vi "Process.vi"(8 "error in":errorcluster, 11 "Inst.AH2500":refnum<class "Inst.AH2500.lvclass">) -> (0 "error out":errorcluster, 3 "Inst.AH2500 out":refnum<class "Inst.AH2500.lvclass">)   [LabVIEW 2019, in "Inst.AH2500.lvclass"]
doc: "---------------------------------------------------------------\nJKI State Machine Objects™\nhttp://jki.net/state-machine-objects/\nCopyright (C) 2005-2015, JKI <info@jki.net>\nALL RIGHTS RESERVED"
uses:
  Inst.AH2500.lvclass
  <vilib>/JKI/JKI SMO/SMO/SMO.lvclass
  <userlib>/LevyLab/Instrument Framework/Instrument/Instrument.lvclass
  <userlib>/LevyLab/RemoteControl/RemoteControl/Typedefs/Message--Cluster.ctl
  <userlib>/LevyLab/RemoteControl/RemoteControl/RemoteControl.lvclass
  Typedefs/PrivateEvents--Inst.AH2500.MessageToProcess.ctl
  <userlib>/LevyLab/Instrument Framework/Instrument Types/VSource/Instrument.VSource.lvclass
  <userlib>/LevyLab/Instrument Framework/Instrument/API/Instrument.sendMessageToProcess (string).vi
  C:/Program Files (x86)/National Instruments/LabVIEW 2019/user.lib/LevyLab/Instrument Framework/Instrument Types/VSource/Instrument.VSource.lvclass
  C:/Program Files (x86)/National Instruments/LabVIEW 2019/user.lib/LevyLab/Instrument Framework/Instrument/Instrument.lvclass
  C:/Program Files (x86)/National Instruments/LabVIEW 2019/vi.lib/JKI/JKI SMO/SMO/SMO.lvclass
panel:
  out "Status":string
  out "State History":string
  # "Inst.AH2500"
  # "Inst.AH2500"
  # "For instructions on how to use the JKI State Machine Objects, examples and video tutorials, visit:\nhttp://jki.net/state-machine-objects/\n\nJKI State Machine Objects™\nhttp://jki.net/state-machine-objects/\nCopyright (C) 2005-2015, JKI <info@jki.net>\nALL RIGHTS RESERVED"
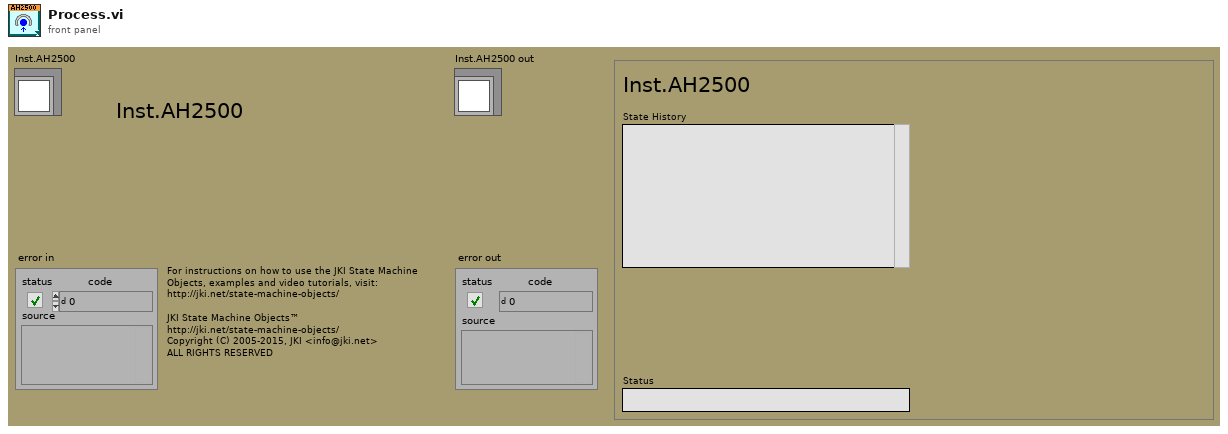
[diagram p1: front panel]
types:
  T1 = enum32{"invalid app kind", "Development System", "Run Time System", "Student Edition", "Embedded LabVIEW", "Evaluation", "Custom"}
  T2 = enum32{"Invalid", "Standard", "Closed", "Hidden", "Minimized", "Maximized"}
  T3 = typedef "RemoteControl.lvclass/Message--Cluster.ctl" = cluster{"Command":string, "Data":variant, "ID":string}
  T4 = typedef "Inst.AH2500.lvclass/PrivateEvents--Inst.AH2500.MessageToProcess.ctl" = cluster{"Message":T5}
  T5 = typedef "RemoteControl.lvlib/RemoteControl.lvclass/Message--Cluster.ctl" = cluster{"Command":string, "Data":variant, "ID":string}
  T6 = cluster{"Core":cluster{"Current VI Reference":refnum<vi>, "Close Panel on Exit?":bool, "Last Error":cluster{"error":errorcluster, "previous state":string, "remaining states":string}, "Shutdown?":bool}, "SelfRef":refnum<class "Inst.AH2500.lvclass">, "Running Step":i32, "sequence":string[], "MessageToProcess":T4}
  T7 = cluster{"Current VI Reference":refnum<vi>, "Close Panel on Exit?":bool, "Last Error":cluster{"error":errorcluster, "previous state":string, "remaining states":string}, "Shutdown?":bool}
  T8 = typedef "smo.lvlib/SMO.lvclass/Protected Events.ctl" = cluster{"StopProcesses":refnum<user-event>, "AbortProcesses":refnum<user-event>, "Config Changed":refnum<user-event>, "Dependency":refnum<user-event>}
  T9 = typedef "Inst.AH2500.lvclass/Inst.AH2500.getAll--Cluster.ctl" = cluster{"capacitance (pF)":dbl, "loss (nS)":dbl, "Vexc (V)":dbl}
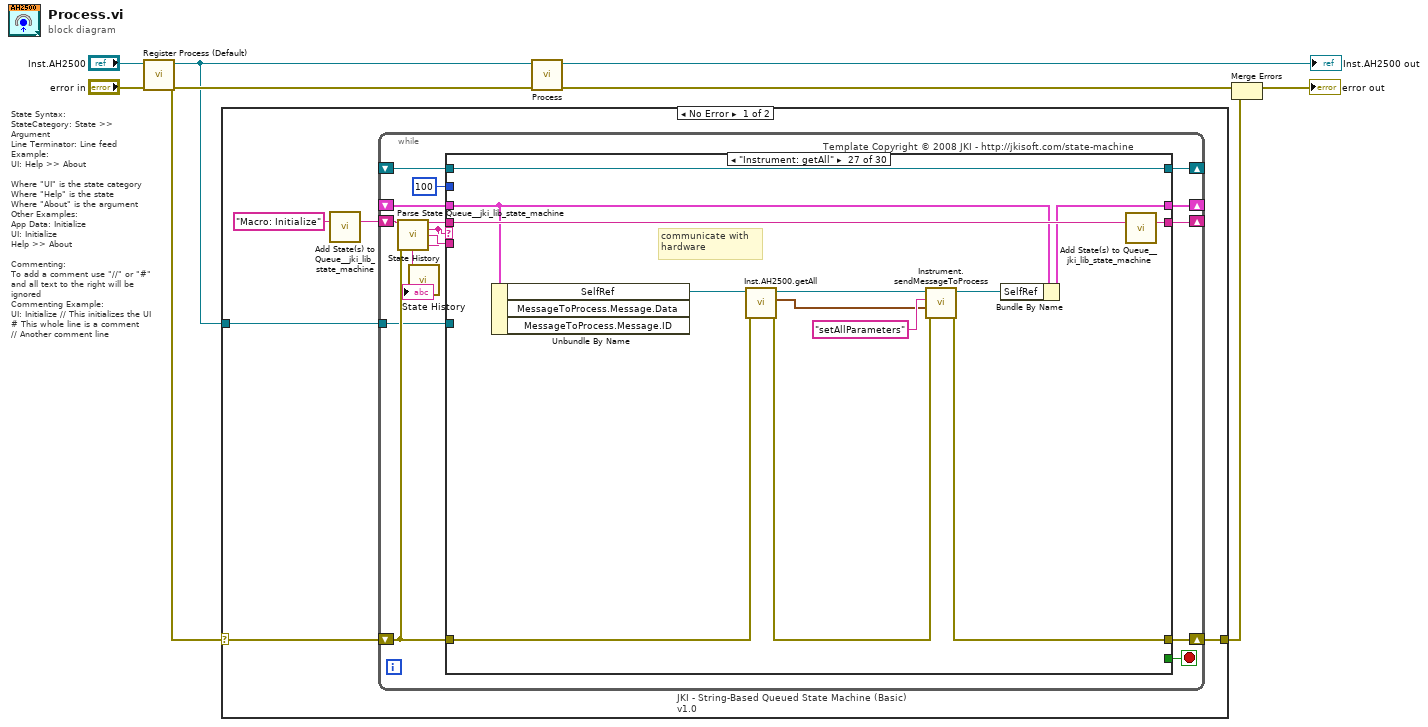
[diagram p0: block diagram]
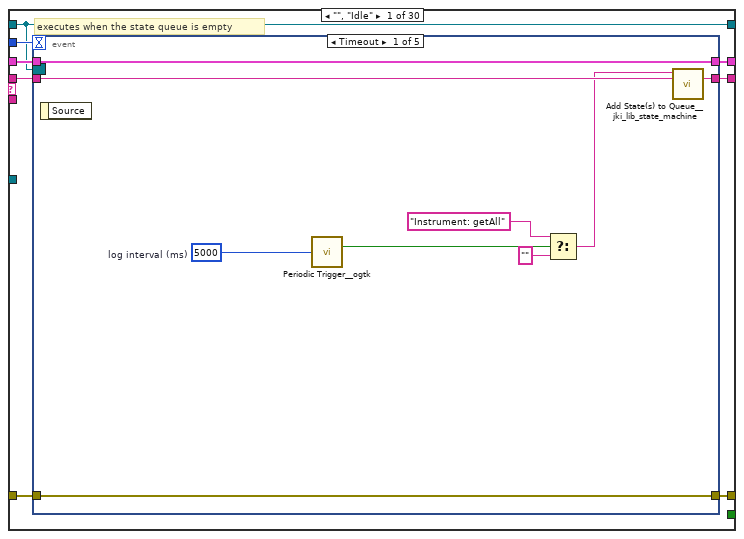
[diagram p2: hidden frame]
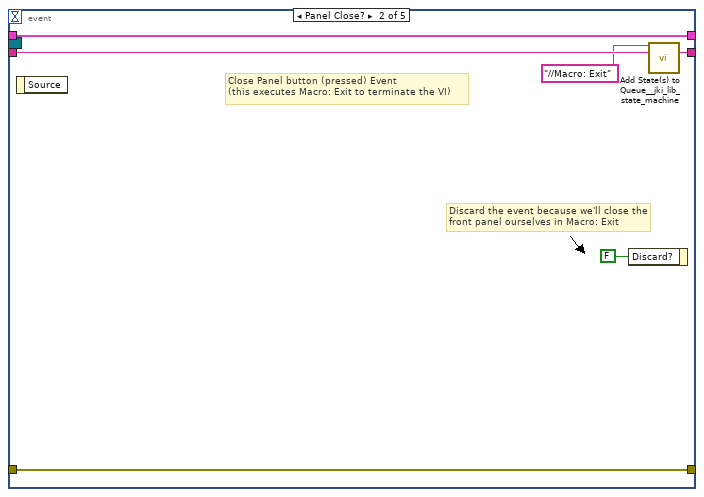
[diagram p3: hidden frame]
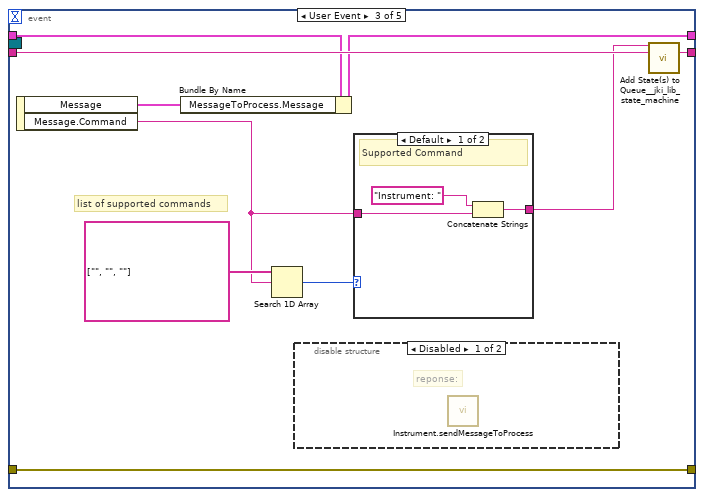
[diagram p4: hidden frame]
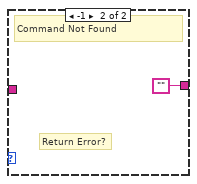
[diagram p6: hidden frame]
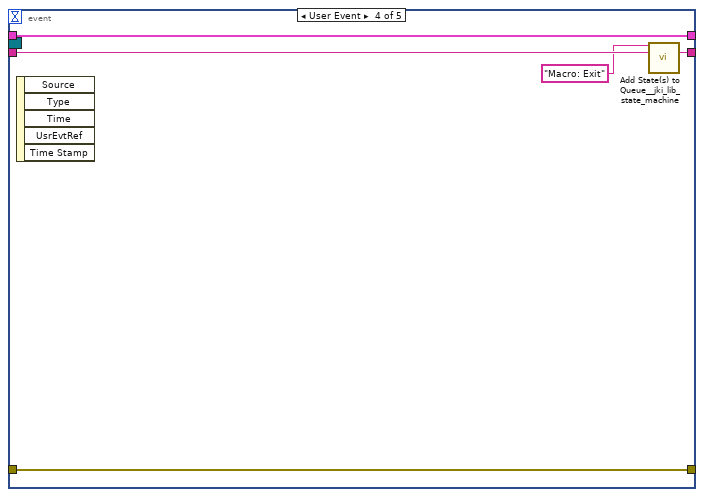
[diagram p7: hidden frame]
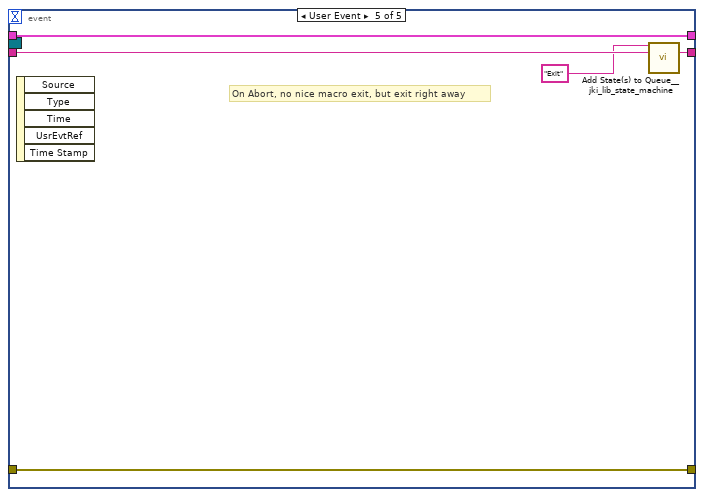
[diagram p8: hidden frame]
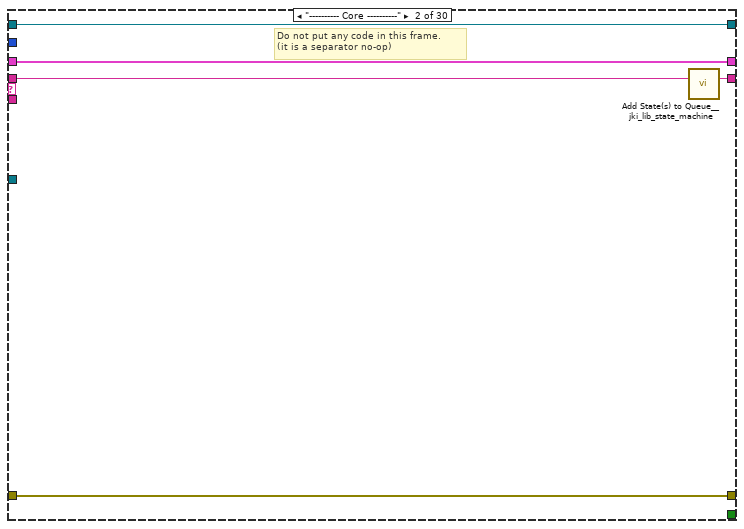
[diagram p9: hidden frame]
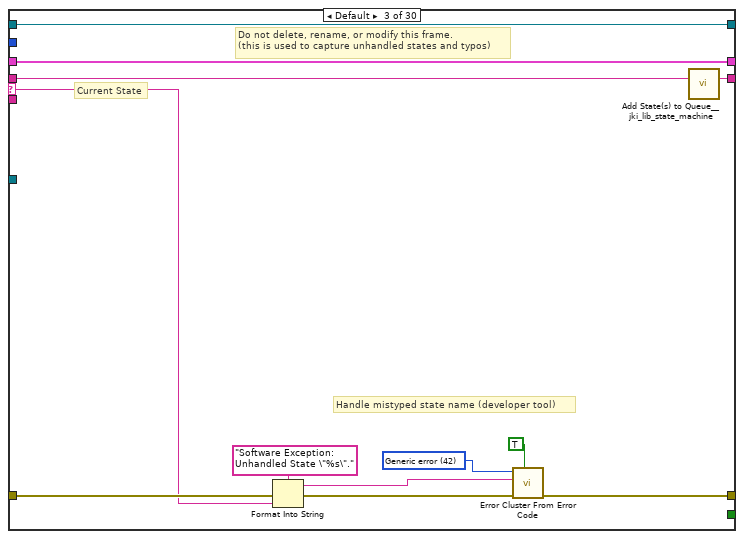
[diagram p10: hidden frame]
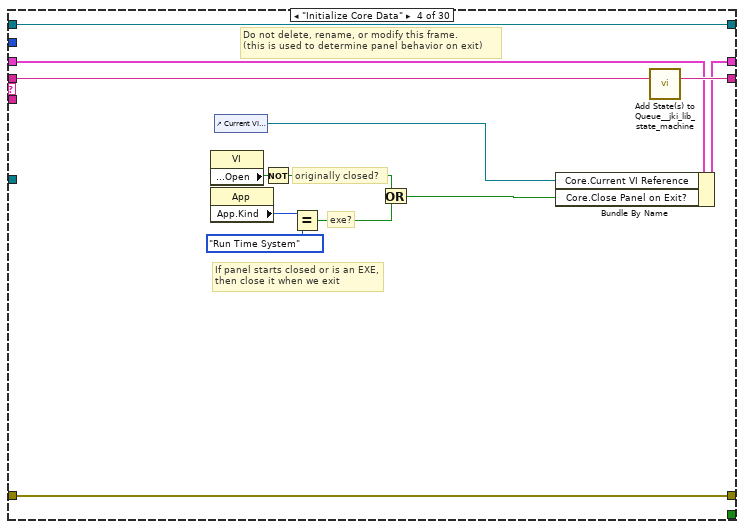
[diagram p11: hidden frame]
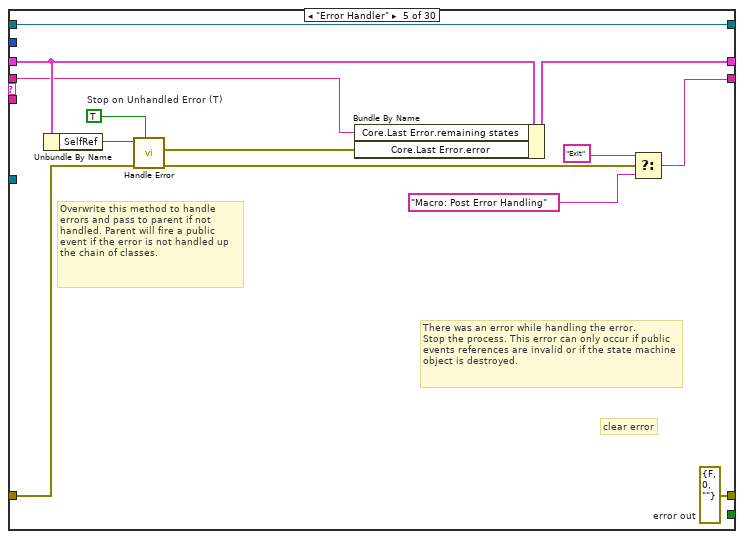
[diagram p12: hidden frame]
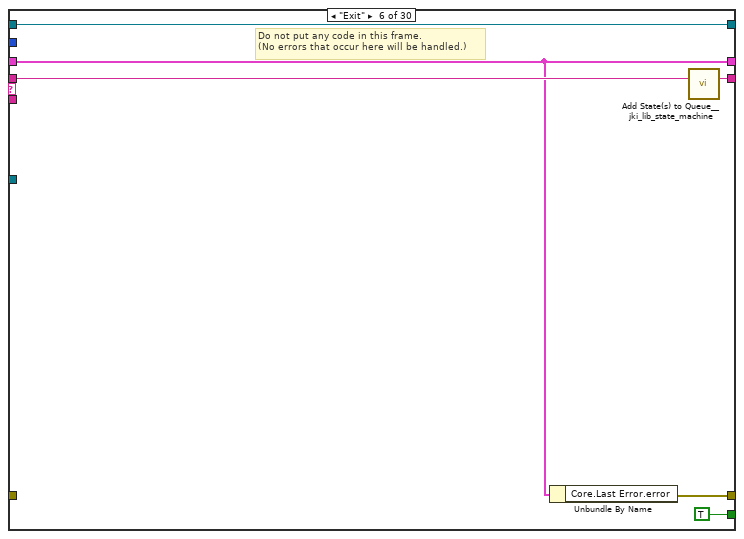
[diagram p13: hidden frame]
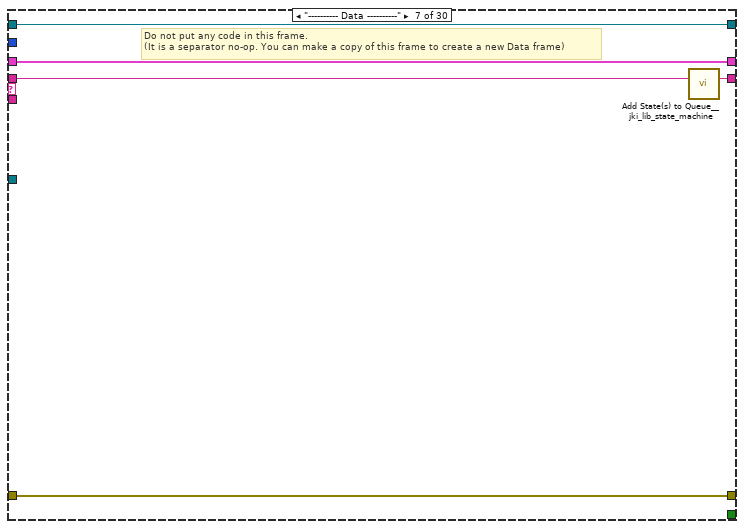
[diagram p14: hidden frame]
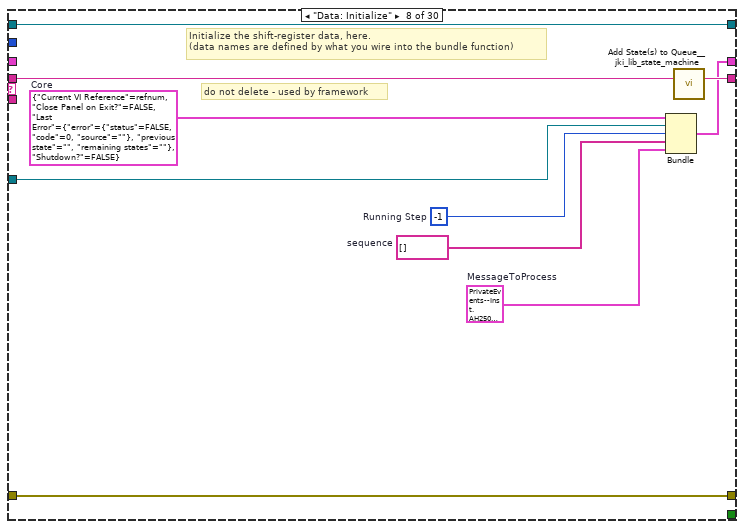
[diagram p15: hidden frame]
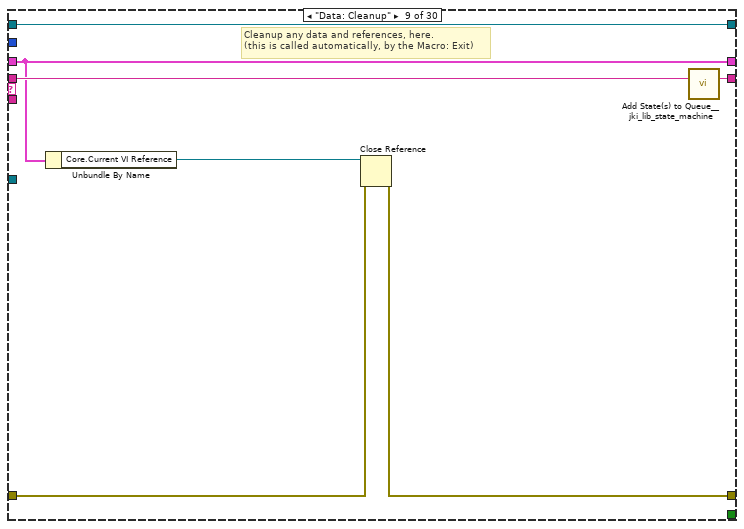
[diagram p16: hidden frame]
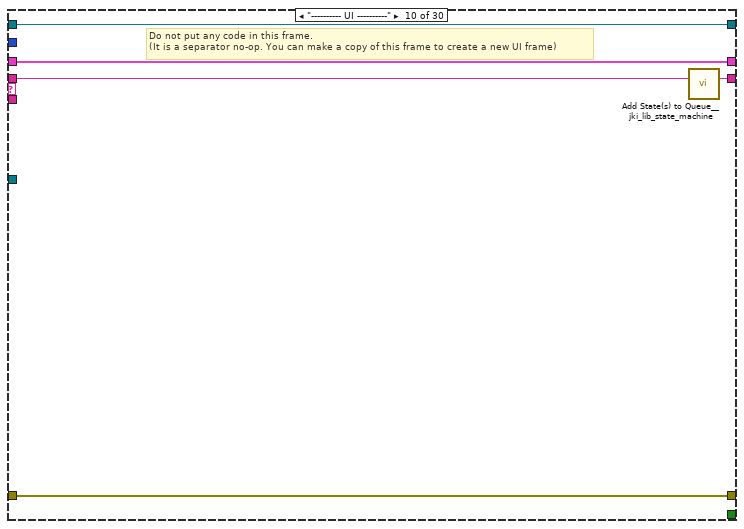
[diagram p17: hidden frame]
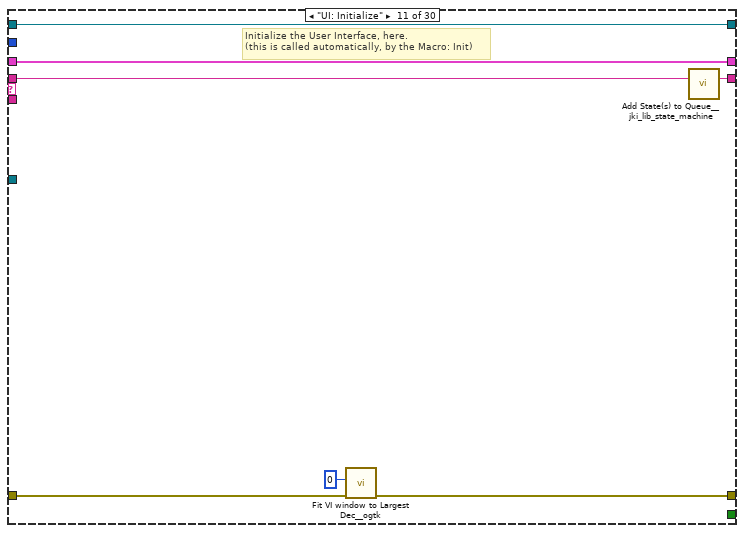
[diagram p18: hidden frame]
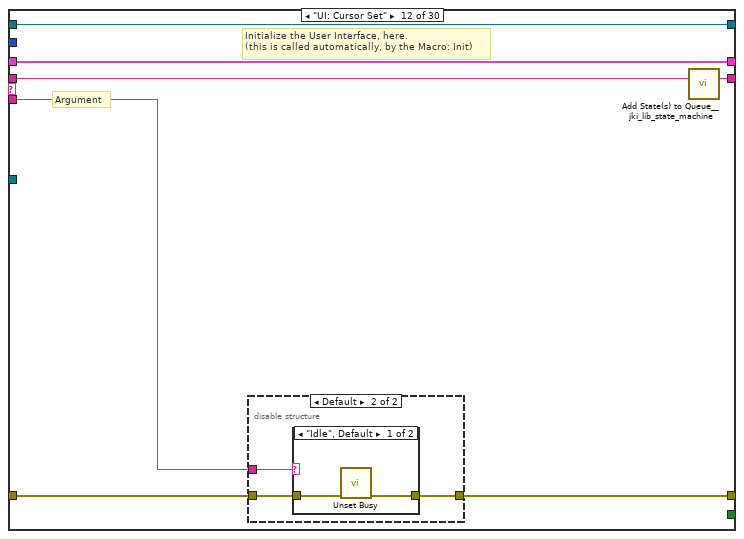
[diagram p19: hidden frame]
diagram:
  # "State Syntax:\nStateCategory: State >> Argument\nLine Terminator: Line feed\nExample:\nUI: Help >> About\n\nWhere \"UI\" is the state category\nWhere \"Help\" is the state\nWhere \"About\" is the argument\nOther Examples:\nApp Data: Initialize\nUI: Initialize\nHelp >> About\n\nCommenting:\nTo add a comment use \"//\" or \"#\" and all text to the right will be ignored\nCommenting Example:\nUI: Initialize // This initializes the UI\n# This whole line is a comment\n// Another comment line"
  n1 = call <vilib>:"Register Process (Default).vi"("error in (no error)"="error in", "SMO"="Inst.AH2500") -> ("error out"=w5:errorcluster, "SelfRef"=w4:refnum<class "Inst.AH2500.lvclass">)  [unwired: 8 in]
  n2 = case shown="No Error" w5 {
    selector: w5 -> [w10 w396]
    tunnel: w4 -> [w11 _]
    tunnel: [w9 w396] -> w1
    frame No Error {
      n3 = call <vilib>:"Add State(s) to Queue__jki_lib_state_machine.vi"("State(s) in (\"\")"="Macro: Initialize") -> ("States Out"=w13:string)  [unwired: 14 in]
      n4 = while "JKI - String-Based Queued State Machine (Basic) v1.0" {
        shift-right: [w22] -> _
        shift-left: _ -> [w21]
        shift-right: [w25] -> w9
        shift-left: w10 -> [w19]
        shift-right: [w24] -> _
        shift-left: w13 -> [w26]
        tunnel: w11 -> [w18]
        shift-right: [w17] -> _
        shift-left: _ -> [w16]
        stop <- w23 stop-if-true
        # "Template Copyright © 2008 JKI - http://jkisoft.com/state-machine"
        n5 = call <vilib>:"Parse State Queue__jki_lib_state_machine.vi"("State Queue"=w26, "Error In (no error)"=w19) -> ("Remaining States"=w28:string, "Current State"=w15:string, "Arguments"=w27:string)  [unwired: 11 in]
        n6 = call <userlib>:"State History.vi"("Current State"=w15) -> ("History"=→"State History":string)  [unwired: 10 in]
        n7 = case shown="\"Instrument: getAll\"" w15 {
          selector: w15 -> [_ _ w82 _ _ _ _ _ _ _ _ _ _ _ _ _ _ _ _ _ _ _ _ _ _ _ _ _ _ _]
          tunnel: w28 -> [w36 w80 w86 w105 w110 w124 w129 w139 w146 w151 w158 w165 w181 w213 w232 w244 w265 w287 w292 w303 w308 w321 w327 w334 w343 w352 w365 w370 w376 w395]
          tunnel: w27 -> [_ _ _ _ _ _ _ _ _ _ _ w159 w175 _ _ _ _ _ _ _ _ _ _ _ _ _ _ _ w371 w379]
          tunnel: w21 -> [w34 w77 w84 w96 w114 w120 w126 _ w141 w148 w156 w163 w177 w210 w229 w234 w255 w268 w289 w300 w305 w314 w325 w329 w339 w348 w361 w366 w372 w385]
          tunnel: [w33 w78 w88 w102 w115 w119 w127 w131 w142 w149 w153 w160 w178 w211 w217 w242 w263 w270 w290 w294 w306 w317 w323 w331 w336 w345 w355 w367 w373 w387] -> w25
          tunnel: w19 -> [w32 w78 w87 w102 w116 _ w127 w131 w143 w149 w152 w161 w179 w211 w221 w242 w263 w271 w290 w295 w306 w311 w323 w331 w335 w344 w359 w367 w373 w381]
          tunnel: [w35 w79 w85 w104 w106 w123 w128 w138 w145 w150 w157 w164 w180 w212 w231 w243 w264 w286 w291 w302 w307 w320 w326 w333 w342 w351 w364 w369 w375 w394] -> w24
          tunnel: [_ _ _ _ _ TRUE _ _ _ _ _ _ _ _ _ _ _ _ _ _ _ _ _ _ _ _ _ _ _ _] -> w23
          tunnel: [w31 w77 w84 w103 w113 w120 w126 w137 w141 w148 w156 w163 w177 w210 w229 w235 w256 w268 w289 w300 w305 w314 w325 w330 w340 w349 w362 w366 w372 w384] -> w22
          tunnel: 100 ("Timeout") -> [w30 _ _ _ _ _ _ _ _ _ _ _ _ _ _ _ _ _ _ _ _ _ _ _ _ _ _ _ _ _]
          tunnel: w18 -> [_ _ _ _ _ _ _ w132 _ _ _ _ _ _ w225 _ _ w267 _ _ _ _ _ _ _ _ _ _ _ _]
          tunnel: [w29 w76 w81 w93 w118 w121 w125 w136 w140 w147 w155 w162 w174 w209 w230 w241 w262 w281 w288 w301 w304 w319 w324 w332 w341 w350 w363 w368 w374 w393] -> w17
          tunnel: w16 -> [w29 w76 w81 w93 w118 w121 w125 w136 w140 w147 w155 w162 w174 w209 w230 w241 w262 w281 w288 w301 w304 _ w324 w332 w341 w350 w363 w368 w374 w393]
          frame "", "Idle" {
            # "executes when the state queue is empty"
            n8 = event shown="[0] Timeout" {
              selector: w29 -> [_ _ _ _ _]
              dyn-events: _ -> [_ _ _ _ _]
              timeout: w30 -> [_ _ _ _ _]
              tunnel: w36 -> [w45 w51 w61 w70 w75]
              tunnel: [w44 w50 w60 w69 w74] -> w35
              tunnel: w34 -> [w42 w48 w53 w67 w72]
              tunnel: [w43 w49 w59 w68 w73] -> w33
              tunnel: w32 -> [w43 w49 w59 w68 w73]
              tunnel: [w42 w48 w54 w67 w72] -> w31
              event Timeout {
                w39 = u32 5000  # log interval (ms)
                n9 = event-data() -> ()  [unwired: 1 in, 1 out]
                n10 = call <userlib>:"Periodic Trigger__ogtk.vi"("time (ms)"=w39) -> ("Triggered"=w41:bool)  [unwired: 12 in, 2 out]
                n11 = Select(t="Instrument: getAll", s=w41, f="") -> (s? t:f=w38:string)
                n12 = call <vilib>:"Add State(s) to Queue__jki_lib_state_machine.vi"("State(s) in Front (\"\")"=w38, "State(s) in (\"\")"=w45) -> ("States Out"=w44:string)  [unwired: 13 in]
              }
              event Panel Close? {
                # "Discard the event because we'll close the front panel ourselves in Macro: Exit"
                # "Close Panel button (pressed) Event\n(this executes Macro: Exit to terminate the VI)"
                n13 = event-data() -> ()  [unwired: 1 in, 1 out]
                n14 = event-data("Discard?"=FALSE) -> ()  [unwired: 1 in, 1 out]
                n15 = call <vilib>:"Add State(s) to Queue__jki_lib_state_machine.vi"("State(s) in Front (\"\")"="//Macro: Exit", "State(s) in (\"\")"=w51) -> ("States Out"=w50:string)  [unwired: 13 in]
              }
              event User Event {
                # "list of supported commands"
                n16 = event-data() -> ("Message"=w52:T3, "Message.Command"=w55:string)  [unwired: 1 in]
                n17 = Bundle By Name(cluster=w53, "MessageToProcess.Message"=w52) -> (w54:T6)
                n18 = Search 1D Array(1D array=string[] ["", "", ""], element=w55) -> (index of element=w58:i32)  [unwired: 1 in]
                n19 = disable-structure shown="Disabled" {
                  frame Disabled {
                    # "reponse:"
                    n20 = call-poly <userlib>:"Instrument.sendMessageToProcess.vi"() -> ()  [unwired: 10 in, 2 out]
                  }
                  frame Enabled {
                  }
                }
                n21 = case shown="Default" w58 {
                  tunnel: [w64 "" ("Empty String Constant")] -> w56
                  tunnel: w55 -> [w63 _]
                  frame Default {
                    # "Supported Command"
                    n22 = Concatenate Strings("Instrument: ", w63) -> (w64:string)
                  }
                  frame -1 {
                    # "Return Error?"
                    # "Command Not Found"
                  }
                }
                n23 = call <vilib>:"Add State(s) to Queue__jki_lib_state_machine.vi"("State(s) in Front (\"\")"=w56, "State(s) in (\"\")"=w61) -> ("States Out"=w60:string)  [unwired: 13 in]
              }
              event User Event {
                n24 = event-data() -> ()  [unwired: 1 in, 5 out]
                n25 = call <vilib>:"Add State(s) to Queue__jki_lib_state_machine.vi"("State(s) in Front (\"\")"="Macro: Exit", "State(s) in (\"\")"=w70) -> ("States Out"=w69:string)  [unwired: 13 in]
              }
              event User Event {
                # "On Abort, no nice macro exit, but exit right away"
                n26 = event-data() -> ()  [unwired: 1 in, 5 out]
                n27 = call <vilib>:"Add State(s) to Queue__jki_lib_state_machine.vi"("State(s) in Front (\"\")"="Exit", "State(s) in (\"\")"=w75) -> ("States Out"=w74:string)  [unwired: 13 in]
              }
            }
          }
          frame "---------- Core ----------" {
            # "Do not put any code in this frame.\n(it is a separator no-op)"
            n28 = call <vilib>:"Add State(s) to Queue__jki_lib_state_machine.vi"("State(s) in (\"\")"=w80) -> ("States Out"=w79:string)  [unwired: 14 in]
          }
          frame Default {
            w91 = 42 items=["No error", "Argument error", "Memory is full", "Out of zone", "End of file", "File already open", "Generic file I/O error", "File not found", "File permission error", "Disk is full", "Duplicate path", "Too many files open", "System feature not enabled", "Resource file not found", "Cannot add resource", "Resource not found", "Image not found", "Image memory error", "Pen does not exist", "Config type invalid", "Config token not found", "Config parse error", "Config memory error", "Bad external code format", "Bad external code offset", "External code not present", "Null window", "Destroy window error", "Null menu", "Print aborted", "Bad print record", "Print driver error", "Windows error during printing", "Memory error during printing", "Print dialog error", "Generic print error", "Invalid device refnum", "Device not found", "Device parameter error", "Device unit error", "Cannot open device", "Device call aborted", "Generic error", "Cancelled by user", "Object ID too low", "Object ID too high", "Object not in heap", "Unknown heap", "Unknown object (invalid DefProc)", "Unknown object (DefProc not in table)", "Message out of range", "Invalid (null) method", "Unknown message", "Manager call not supported", "Bad address", "Network operation in progress", "Network operation timed out", "Connection is busy", "Network attribute not supported", "Network error", "Address in use", "System out of memory", "Connection aborted", "Connection refused", "Not connected", "Already connected", "Connection closed", "Initialization error (interapplication manager)", "Bad occurrence", "Wait on unbound occurrence handler", "Occurrence queue overflow", "Datalog type conflict", "Unused", "Unrecognized type (interapplication manager)", "Memory corrupt", "Failed to make temporary DLL", "Old CIN version", "Drag socket not found", "Failed to load drop-object", "Failed to register OLE object", "Failed to release OLE object", "Format specifier type mismatch", "Unknown format specifier", "Too few format specifiers", "Too many format specifiers", "Scan failed", "Newer CIN version", "Error converting to variant", "Runtime menu error", "Password tampered", "Variant attribute not found", "Incompatible variant data type", "Event data is not available", "Event Store is not present", "Occurrence is not found", "Event Queue is not created", "Event info is not available", "Refnum passed is NULL", "Error retrieving Class GUID", "Error retrieving CoClass GUID", "Error retrieving TypeLib GUID.", "Bad built application magic bytes.", "Specific driver is different from the specific driver associated with the Logical Name.", "There is no session opened to the class driver.", "Max Error", "MAX - Error with config objects", "MAX - Error loading configuration", "MAX - Group not supported"]
            # "Current State"
            # "Do not delete, rename, or modify this frame.\n(this is used to capture unhandled states and typos)"
            # "Handle mistyped state name (developer tool)"
            n29 = Format Into String(format string="Software Exception: Unhandled State \"%s\"." ("message"), error in=w87, w82) -> (resulting string=w90:string, error out=w89:errorcluster)  [unwired: 1 in]
            n30 = call <vilib>:"Error Cluster From Error Code.vi"("show call chain? (False)"=TRUE, "error in (no error)"=w89, "error message (\"\")"=w90, "error code (0)"=w91) -> ("error out"=w88:errorcluster)  [unwired: 5 in]
            n31 = call <vilib>:"Add State(s) to Queue__jki_lib_state_machine.vi"("State(s) in (\"\")"=w86) -> ("States Out"=w85:string)  [unwired: 14 in]
          }
          frame "Initialize Core Data" {
            # "Do not delete, rename, or modify this frame.\n(this is used to determine panel behavior on exit)"
            # "originally closed?"
            # "exe?"
            # "If panel starts closed or is an EXE, then close it when we exit"
            n32 = property class="VI"() -> ("Front Panel.Open"=w101:bool)  [unwired: 2 in, 2 out]
            n33 = property class="App"() -> ("App.Kind"=w100:T1)  [unwired: 2 in, 2 out]
            n34 = control-ref of="Current VI Reference"() -> (w94:refnum<vi>)
            n35 = Not(x=w101) -> (.not. x?=w98:bool)
            n36 = Equal?(x=w100, y=T1."Run Time System" ("Application:Kind")) -> (x = y?=w97:bool)
            n37 = Or(x=w98, y=w97) -> (x .or. y?=w95:bool)
            n38 = Bundle By Name(cluster=w96, "Core.Current VI Reference"=w94, "Core.Close Panel on Exit?"=w95) -> (w103:T6)
            n39 = call <vilib>:"Add State(s) to Queue__jki_lib_state_machine.vi"("State(s) in (\"\")"=w105) -> ("States Out"=w104:string)  [unwired: 14 in]
          }
          frame "Error Handler" {
            w111 = TRUE  # Stop on Unhandled Error (T)
            w115 = errorcluster {"status"=FALSE, "code"=0, "source"=""}  # error out
            # "clear error"
            # "There was an error while handling the error.\nStop the process. This error can only occur if public events references are invalid or if the state machine object is destroyed."
            # "Overwrite this method to handle errors and pass to parent if not handled. Parent will fire a public event if the error is not handled up the chain of classes."
            n40 = Unbundle By Name(w114) -> ("SelfRef"=w117:refnum<class "Inst.AH2500.lvclass">)
            n41 = call-dynamic "Handle Error.vi"("Stop on Unhandled Error (T)"=w111, "error in"=w116, "SMO"=w117) -> ("handling error"=w107:errorcluster, "Unhandled error"=w112:errorcluster)  [unwired: 6 in, 1 out]
            n42 = Bundle By Name(cluster=w114, "Core.Last Error.remaining states"=w110, "Core.Last Error.error"=w112) -> (w113:T6)
            n43 = Select(t="Exit", s=w107, f="Macro: Post Error Handling") -> (s? t:f=w106:string)
          }
          frame "Exit" {
            # "Do not put any code in this frame.\n(No errors that occur here will be handled.)"
            n44 = Unbundle By Name(w120) -> ("Core.Last Error.error"=w119:errorcluster)
            n45 = call <vilib>:"Add State(s) to Queue__jki_lib_state_machine.vi"("State(s) in (\"\")"=w124) -> ("States Out"=w123:string)  [unwired: 14 in]
          }
          frame "---------- Data ----------" {
            # "Do not put any code in this frame.\n(It is a separator no-op. You can make a copy of this frame to create a new Data frame)"
            n46 = call <vilib>:"Add State(s) to Queue__jki_lib_state_machine.vi"("State(s) in (\"\")"=w129) -> ("States Out"=w128:string)  [unwired: 14 in]
          }
          frame "Data: Initialize" {
            w130 = T4 {"Message"={"Command"="", "Data"=variant(string ""), "ID"=""}}  # MessageToProcess
            w133 = string[] []  # sequence
            w134 = -1  # Running Step
            w135 = T7 {"Current VI Reference"=refnum, "Close Panel on Exit?"=FALSE, "Last Error"={"error"={"status"=FALSE, "code"=0, "source"=""}, "previous state"="", "remaining states"=""}, "Shutdown?"=FALSE}  # Core
            # "do not delete - used by framework"
            # "Initialize the shift-register data, here.\n(data names are defined by what you wire into the bundle function)"
            n47 = Bundle("Core"=w135, "SelfRef"=w132, "Running Step"=w134, "sequence"=w133, "MessageToProcess"=w130) -> (w137:T6)  [unwired: 1 in]
            n48 = call <vilib>:"Add State(s) to Queue__jki_lib_state_machine.vi"("State(s) in (\"\")"=w139) -> ("States Out"=w138:string)  [unwired: 14 in]
          }
          frame "Data: Cleanup" {
            # "Cleanup any data and references, here.\n(this is called automatically, by the Macro: Exit)"
            n49 = Unbundle By Name(w141) -> ("Core.Current VI Reference"=w144:refnum<vi>)
            n50 = Close Reference(reference=w144, error in (no error)=w143) -> (error out=w142:errorcluster)
            n51 = call <vilib>:"Add State(s) to Queue__jki_lib_state_machine.vi"("State(s) in (\"\")"=w146) -> ("States Out"=w145:string)  [unwired: 14 in]
          }
          frame "---------- UI ----------" {
            # "Do not put any code in this frame.\n(It is a separator no-op. You can make a copy of this frame to create a new UI frame)"
            n52 = call <vilib>:"Add State(s) to Queue__jki_lib_state_machine.vi"("State(s) in (\"\")"=w151) -> ("States Out"=w150:string)  [unwired: 14 in]
          }
          frame "UI: Initialize" {
            # "Initialize the User Interface, here.\n(this is called automatically, by the Macro: Init)"
            n53 = call <userlib>:"Fit VI window to Largest Dec__ogtk.vi"("error in (no error)"=w152, "border spacing (2 px)"=0) -> ("error out"=w153:errorcluster)  [unwired: 4 in, 1 out]
            n54 = call <vilib>:"Add State(s) to Queue__jki_lib_state_machine.vi"("State(s) in (\"\")"=w158) -> ("States Out"=w157:string)  [unwired: 14 in]
          }
          frame "UI: Cursor Set" {
            # "Argument"
            # "Initialize the User Interface, here.\n(this is called automatically, by the Macro: Init)"
            n55 = disable-structure shown="Default" {
              disable-tunnel: w161 -> [w166 w169]
              disable-tunnel: [w166 w168] -> w160
              disable-tunnel: w159 -> [_ w167]
              frame condition #0 {
              }
              frame condition #1 (active) {
                n56 = case shown="\"Idle\", Default" w167 {
                  tunnel: w169 -> [w171 w173]
                  tunnel: [w170 w172] -> w168
                  frame "Idle", Default {
                    n57 = call <vilib>:"Unset Busy.vi"("error in (no error)"=w171) -> ("error out"=w170:errorcluster)  [unwired: 10 in]
                  }
                  frame "Busy" {
                    n58 = call <vilib>:"Set Busy.vi"("error in (no error)"=w173) -> ("error out"=w172:errorcluster)  [unwired: 9 in, 1 out]
                  }
                }
              }
            }
            n59 = call <vilib>:"Add State(s) to Queue__jki_lib_state_machine.vi"("State(s) in (\"\")"=w165) -> ("States Out"=w164:string)  [unwired: 14 in]
          }
          frame "UI: Front Panel State" {
            # "Argument"
            # "Set Front Panel Open or Closed\n(Usage: \"UI: Front Panel State >> Open|Close\")"
            n60 = Unbundle By Name(w177) -> ("Core.Current VI Reference"=w176:refnum<vi>)
            n61 = disable-structure shown="TARGET_TYPE==RT" {
              disable-tunnel: w179 -> [w185 w208]
              disable-tunnel: [w184 w208] -> w178
              disable-tunnel: w176 -> [w183 _]
              disable-tunnel: w175 -> [w182 _]
              frame condition #0 (active) {
                n62 = case shown="\"Close\"" w182 {
                  tunnel: w185 -> [w189 w202]
                  tunnel: [w191 w203] -> w184
                  tunnel: w183 -> [w190 w200]
                  frame "Open", Default {
                    n63 = property class="VI"(reference=w190, error in=w189) -> (reference out=w187:refnum<vi>, error out=w188:errorcluster, "FP.State"=w186:T2)
                    n64 = case shown="\"Closed\"" w186 {
                      tunnel: [w194 w197] -> w191
                      tunnel: w188 -> [w193 w197]
                      tunnel: w187 -> [w192 _]
                      frame "Closed" {
                        n65 = invoke class="VI" method="FP.Open"(reference=w192, error in=w193, "Activate"=TRUE, "State"=T2."Standard") -> (error out=w194:errorcluster)  [unwired: 1 in, 4 out]
                      }
                      frame Default {
                      }
                    }
                  }
                  frame "Close" {
                    n66 = property class="VI"(reference=w200, error in=w202) -> (reference out=w199:refnum<vi>, error out=w201:errorcluster, "FP.State"=w198:T2)
                    n67 = case shown="Default" w198 {
                      tunnel: [w204 w207] -> w203
                      tunnel: w201 -> [w204 w206]
                      tunnel: w199 -> [_ w205]
                      frame "Invalid", "Closed" {
                      }
                      frame Default {
                        n68 = invoke class="VI" method="FP.Close"(reference=w205, error in=w206) -> (error out=w207:errorcluster)  [unwired: 1 in, 2 out]
                      }
                    }
                  }
                }
              }
              frame condition #1 {
              }
            }
            n69 = call <vilib>:"Add State(s) to Queue__jki_lib_state_machine.vi"("State(s) in (\"\")"=w181) -> ("States Out"=w180:string)  [unwired: 14 in]
          }
          frame "---------- Macro ----------" {
            # "Do not put any code in this frame.\n(It is a separator no-op. You can make a copy of this frame to create a new Macro frame)"
            n70 = call <vilib>:"Add State(s) to Queue__jki_lib_state_machine.vi"("State(s) in (\"\")"=w213) -> ("States Out"=w212:string)  [unwired: 14 in]
          }
          frame "Macro: Initialize" {
            # "Initialization Macro\n(This is called once, when the VI starts)"
            n71 = call-dynamic "Read Debug Mode.vi"("error in (no error)"=w221, "Instrument in"=w225) -> ("error out"=w220:errorcluster, "Debug Mode?"=w222:bool)  [unwired: 7 in, 1 out]
            n72 = call <userlib>:"Wait (ms)__ogtk.vi"("error in (no error)"=w220, "milliseconds to wait"=u32 0) -> ("error out"=w217:errorcluster)  [unwired: 8 in, 1 out]
            n73 = Select(t="Open", s=w222, f="Close") -> (s? t:f=w218:string)
            n74 = Format Into String(format string="UI: Initialize\nUI: Front Panel State >> %s\nInstrument: Open Hardware", initial string="", w218) -> (resulting string=w219:string)  [unwired: 1 in, 1 out]
            n75 = call <vilib>:"Add State(s) to Queue__jki_lib_state_machine.vi"("State(s) in Front (\"\")"="Data: Initialize\nInitialize Core Data\nEvents: Register", "State(s) in (\"\")"="Process: Sync", "State(s) at Back (\"\")"=w219) -> ("States Out"=w227:string)  [unwired: 12 in]
            n76 = call <vilib>:"Add State(s) to Queue__jki_lib_state_machine.vi"("State(s) in Front (\"\")"=w227, "State(s) in (\"\")"=w232) -> ("States Out"=w231:string)  [unwired: 13 in]
          }
          frame "Macro: Post Error Handling" {
            # "Clear Last Error?"
            n77 = Unbundle By Name(w234) -> ("Core.Last Error.remaining states"=w236:string, "Core.Shutdown?"=w237:bool)
            n78 = Unbundle By Name(w234) -> ("Core.Last Error.error"=w240:errorcluster)
            n79 = case shown="False" FALSE {
              tunnel: w240 -> [w248 _]
              tunnel: [w248 _] -> w239
              frame False {
              }
              frame True {
              }
            }
            n80 = case shown="True" w237 {
              tunnel: w236 -> [w245 w247]
              tunnel: [w245 w246] -> w233
              frame False {
                # "These are the remaining states (at the moment the error occured). States can be altered according to business logic."
                # "NOT SHUTTING DOWN"
              }
              frame True {
                # "Developer can decide to alter the states but should be aware that during the shutdown process, there are certain states that must be run for the SMO to properly shut itself (and this process) down. As such, one can add states to perform additional clean-ups, but should append the remaining state to be executed."
                # "SHUTTING DOWN"
                n81 = call <vilib>:"Add State(s) to Queue__jki_lib_state_machine.vi"("State(s) in (\"\")"=w247) -> ("States Out"=w246:string)  [unwired: 14 in]
              }
            }
            n82 = Bundle By Name(cluster=w234, "Core.Last Error.error"=w239) -> (w235:T6)
            n83 = call <vilib>:"Add State(s) to Queue__jki_lib_state_machine.vi"("State(s) in Front (\"\")"=w233, "State(s) in (\"\")"=w244) -> ("States Out"=w243:string)  [unwired: 13 in]
          }
          frame "Macro: Run Sequence" {
            # "0,1,2,3,4,"
            # "5"
            # "Do not put any code in this frame.\n(It is a separator no-op. You can make a copy of this frame to create a new Macro frame)"
            n84 = Unbundle By Name(w255) -> ("sequence"=w251:string[], "Running Step"=w249:i32)
            n85 = Array Size(array=w251) -> (size(s)=w261:i32)
            n86 = Index Array(array=w251, index=w249) -> (element=w250:string)
            n87 = Greater Or Equal?(x=w261, y=w249) -> (x >= y?=w253:bool)
            n88 = Select(t=-1 ("Running Step"), s=w253, f=w249) -> (s? t:f=w260:i32)
            n89 = Bundle By Name(cluster=w255, "Running Step"=w260) -> (w256:T6)
            n90 = Select(t="Sequence: Status >> ...", s=w253, f="Idle //Check Event Structure\nMacro: Run Sequence" ("State(s) at Back (\"\")")) -> (s? t:f=w252:string)
            n91 = call <vilib>:"Add State(s) to Queue__jki_lib_state_machine.vi"("State(s) in Front (\"\")"=w250, "State(s) at Back (\"\")"=w252) -> ("States Out"=w254:string)  [unwired: 13 in]
            n92 = call <vilib>:"Add State(s) to Queue__jki_lib_state_machine.vi"("State(s) in Front (\"\")"=w254, "State(s) in (\"\")"=w265) -> ("States Out"=w264:string)  [unwired: 13 in]
          }
          frame "Macro: Exit" {
            # "Exit Macro\n(This is called once, when the VI exits)"
            n93 = Unbundle By Name(w268) -> ("Core.Close Panel on Exit?"=w285:bool)
            n94 = call-dynamic "Read Debug Mode.vi"("error in (no error)"=w271, "Instrument in"=w267) -> ("error out"=w270:errorcluster, "Debug Mode?"=w269:bool)  [unwired: 7 in, 1 out]
            n95 = Select(t="Open", s=w269, f="Close") -> (s? t:f=w275:string)
            n96 = call <vilib>:"Build State String with Arguments__JKI_lib_State_Machine.vi"("Arguments (\"\")"=w275, "State"="UI: Front Panel State") -> ("State with Arguments"=w272:string)  [unwired: 4 in]
            n97 = Select(t=w272, s=w285, f="" ("Empty String Constant")) -> (s? t:f=w283:string)
            n98 = call <vilib>:"Add State(s) to Queue__jki_lib_state_machine.vi"("State(s) in Front (\"\")"="Data: Cleanup\nEvents: Unregister", "State(s) in (\"\")"="Process: Sync", "State(s) at Back (\"\")"="Exit") -> ("States Out"=w278:string)  [unwired: 12 in]
            n99 = call <vilib>:"Add State(s) to Queue__jki_lib_state_machine.vi"("State(s) in Front (\"\")"="Instrument: Close Hardware", "State(s) in (\"\")"=w283, "State(s) at Back (\"\")"=w278) -> ("States Out"=w282:string)  [unwired: 12 in]
            n100 = call <vilib>:"Add State(s) to Queue__jki_lib_state_machine.vi"("State(s) in Front (\"\")"=w282, "State(s) in (\"\")"=w287) -> ("States Out"=w286:string)  [unwired: 13 in]
          }
          frame "---------- Process ----------" {
            # "Template Separator\n(You can make a copy of, or modify, this frame)"
            n101 = call <vilib>:"Add State(s) to Queue__jki_lib_state_machine.vi"("State(s) in (\"\")"=w292) -> ("States Out"=w291:string)  [unwired: 14 in]
          }
          frame "Process: Sync" {
            n102 = Unbundle By Name(w300) -> ("SelfRef"=w296:refnum<class "Inst.AH2500.lvclass">)
            n103 = call <vilib>:"WaitOnProcessSync.vi"("error in (no error)"=w295, "SMO"=w296) -> ("error out"=w294:errorcluster, "Don't run?"=w299:bool)  [unwired: 7 in, 1 out]
            n104 = Select(t="Data: Cleanup\nEvents: Unregister\nExit", s=w299, f="" ("Empty String Constant")) -> (s? t:f=w293:string)
            n105 = call <vilib>:"Add State(s) to Queue__jki_lib_state_machine.vi"("State(s) in Front (\"\")"=w293, "State(s) in (\"\")"=w303) -> ("States Out"=w302:string)  [unwired: 13 in]
          }
          frame "---------- Events ----------" {
            # "Template Separator\n(You can make a copy of, or modify, this frame)"
            n106 = call <vilib>:"Add State(s) to Queue__jki_lib_state_machine.vi"("State(s) in (\"\")"=w308) -> ("States Out"=w307:string)  [unwired: 14 in]
          }
          frame "Events: Register" {
            n107 = Unbundle By Name(w314) -> ("SelfRef"=w315:refnum<class "Inst.AH2500.lvclass">)
            n108 = call <vilib>:"GetProtectedEvents.vi"("SMO"=w315) -> ("error out"=w313:errorcluster, "SMO Protected Events"=w318:T8, "SMO out"=w312:refnum<class "Inst.AH2500.lvclass">)  [unwired: 8 in]
            n109 = call "Inst.AH2500.GetPrivateEvents.vi"("Inst.AH2500 in"=w312) -> ("error out"=w309:errorcluster, "Inst.AH2500 Private Events"=w310:cluster{"MessageToProcess":refnum<user-event>})  [unwired: 8 in, 1 out]
            n110 = register-events(w318, w310) -> (reference out=w319:refnum<event-registration>, error out=w316:errorcluster)  [unwired: 2 in]
            n111 = Merge Errors(w316, w309, w313, w311) -> (w317:errorcluster)
            n112 = call <vilib>:"Add State(s) to Queue__jki_lib_state_machine.vi"("State(s) in (\"\")"=w321) -> ("States Out"=w320:string)  [unwired: 14 in]
          }
          frame "Events: Unregister" {
            n113 = Unregister For Events(event registration refnum=w324, error in=w323) -> (error out=w322:errorcluster)
            n114 = call <vilib>:"Clear Errors.vi"("error in (no error)"=w322) -> ()  [unwired: 5 in, 2 out]
            n115 = call <vilib>:"Add State(s) to Queue__jki_lib_state_machine.vi"("State(s) in (\"\")"=w327) -> ("States Out"=w326:string)  [unwired: 14 in]
          }
          frame "---------- Instrument ----------" {
            n116 = Unbundle By Name(w329) -> ("SelfRef"=w328:refnum<class "Inst.AH2500.lvclass">)
            n117 = Bundle By Name(cluster=w329, "SelfRef"=w328) -> (w330:T6)
            n118 = call <vilib>:"Add State(s) to Queue__jki_lib_state_machine.vi"("State(s) in (\"\")"=w334) -> ("States Out"=w333:string)  [unwired: 14 in]
          }
          frame "Instrument: Open Hardware" {
            n119 = Unbundle By Name(w339) -> ("SelfRef"=w338:refnum<class "Inst.AH2500.lvclass">)
            n120 = call-dynamic "Open Hardware.vi"("error in (no error)"=w335, "Inst.AH2500 in"=w338) -> ("error out"=w336:errorcluster, "Inst.AH2500 out"=w337:refnum<class "Inst.AH2500.lvclass">)  [unwired: 8 in]
            n121 = Bundle By Name(cluster=w339, "SelfRef"=w337) -> (w340:T6)
            n122 = call <vilib>:"Add State(s) to Queue__jki_lib_state_machine.vi"("State(s) in (\"\")"=w343) -> ("States Out"=w342:string)  [unwired: 14 in]
          }
          frame "Instrument: Close Hardware" {
            n123 = Unbundle By Name(w348) -> ("SelfRef"=w347:refnum<class "Inst.AH2500.lvclass">)
            n124 = call-dynamic "Close Hardware.vi"("error in (no error)"=w344, "Inst.AH2500 in"=w347) -> ("error out"=w345:errorcluster, "Inst.AH2500 out"=w346:refnum<class "Inst.AH2500.lvclass">)  [unwired: 8 in]
            n125 = Bundle By Name(cluster=w348, "SelfRef"=w346) -> (w349:T6)
            n126 = call <vilib>:"Add State(s) to Queue__jki_lib_state_machine.vi"("State(s) in (\"\")"=w352) -> ("States Out"=w351:string)  [unwired: 14 in]
          }
          frame "Instrument: getAll" {
            # "communicate with\nhardware"
            n127 = Unbundle By Name(w361) -> ("SelfRef"=w360:refnum<class "Inst.AH2500.lvclass">)  [unwired: 2 out]
            n128 = call "Inst.AH2500.getAll.vi"("error in (no error)"=w359, "Inst.AH2500 in"=w360) -> ("error out"=w356:errorcluster, "output cluster"=w357:T9, "Inst.AH2500 out"=w354:refnum<class "Inst.AH2500.lvclass">)  [unwired: 7 in]
            n129 = call-poly <userlib>:"Instrument.sendMessageToProcess.vi"("error in (no error)"=w356, "Data"=w357, "Command"="setAllParameters", "Instrument"=w354) -> ("error out"=w355:errorcluster, "Instrument out"=w353:refnum<class "Inst.AH2500.lvclass">)  [unwired: 6 in]
            n130 = Bundle By Name(cluster=w361, "SelfRef"=w353) -> (w362:T6)
            n131 = call <vilib>:"Add State(s) to Queue__jki_lib_state_machine.vi"("State(s) in (\"\")"=w365) -> ("States Out"=w364:string)  [unwired: 14 in]
          }
          frame "---------- Sequence ----------" {
            n132 = call <vilib>:"Add State(s) to Queue__jki_lib_state_machine.vi"("State(s) in (\"\")"=w370) -> ("States Out"=w369:string)  [unwired: 14 in]
          }
          frame "Sequence: Status" {
            # "Sequence: Status\n(Use this frame to pass the status to the UI, this VI's UI, etc)"
            n133 = call <vilib>:"Add State(s) to Queue__jki_lib_state_machine.vi"("State(s) in (\"\")"=w376) -> ("States Out"=w375:string)  [unwired: 14 in]
            "Status" <- w371
          }
          frame "Sequence: Wait" {
            # "Sequence: Wait\n(Non-Blocking Wait)"
            # "F = repeat this state. wait\nT = go to next state. don't wait"
            n134 = Unbundle By Name(w385) -> ("Running Step"=w378:i32)
            n135 = call <userlib>:"Wait Logic.vi"("error in (no error)"=w381, "Time"=w379) -> ("error out"=w380:errorcluster, "Status String"=w377:string, "Trigger"=w382:bool)  [unwired: 6 in, 1 out]
            n136 = Increment(x=w378) -> (x+1=w392:i32)
            n137 = Select(t=w392, s=w382, f=w378) -> (s? t:f=w383:i32)
            n138 = Select(t=u32 0, s=w382, f=u32 100 ("milliseconds to wait")) -> (s? t:f=w389:u32)
            n139 = call <userlib>:"Wait (ms)__ogtk.vi"("error in (no error)"=w380, "milliseconds to wait"=w389) -> ("error out"=w387:errorcluster)  [unwired: 8 in, 1 out]
            n140 = Bundle By Name(cluster=w385, "Running Step"=w383) -> (w384:T6)
            n141 = call <vilib>:"Build State String with Arguments__JKI_lib_State_Machine.vi"("Arguments (\"\")"=w377, "State"="Sequence: Status") -> ("State with Arguments"=w386:string)  [unwired: 4 in]
            n142 = call <vilib>:"Add State(s) to Queue__jki_lib_state_machine.vi"("State(s) in Front (\"\")"=w386, "State(s) in (\"\")"=w395) -> ("States Out"=w394:string)  [unwired: 13 in]
          }
        }
      }
    }
    frame Error {
    }
  }
  n143 = call-parent "Process.vi"("error in"=w5, "Instrument"=w4) -> ("error out"=w2:errorcluster, "Instrument out"=→"Inst.AH2500 out":refnum<class "Inst.AH2500.lvclass">)  [unwired: 8 in]
  n144 = Merge Errors(w2, w1) -> (→"error out":errorcluster)
